vi "DiHuiTech Main.vi"(8 "error in (no error)":errorcluster caption="错误输入（无错误）", 10 "枚举":T3, 11 "Temperature&Humidity":T2) -> (0 "错误输出":errorcluster, 2 "value":T1, 3 "result":bool)   [LabVIEW 2017]
uses:
  DiHuiTech Operation.ctl
  DiHuiTech Param.ctl
  DiHuiTech Value.ctl
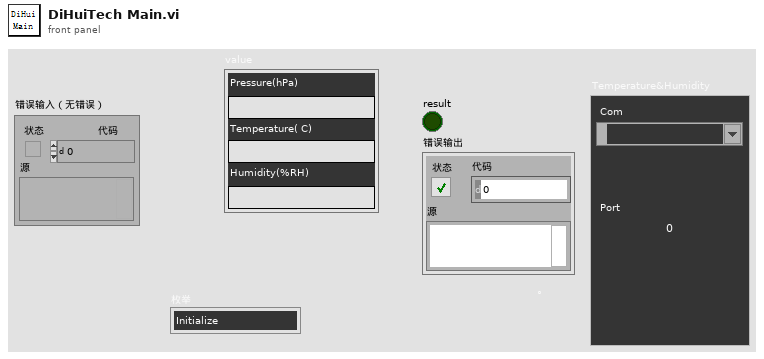
[diagram p1: front panel]
types:
  T1 = typedef "DiHuiTech Value.ctl" = cluster{"Pressure(hPa)":string, "Temperature( C)":string, "Humidity(%RH)":string}
  T2 = typedef "DiHuiTech Param.ctl" = cluster{"Com":refnum<visa-resource-name>, "Port":u32}
  T3 = typedef "DiHuiTech Operation.ctl" = enum16{"Initialize", "Read", "Exit"}
  T4 = cluster{"Pressure":dbl, "Temperature":dbl, "Humidity":dbl}
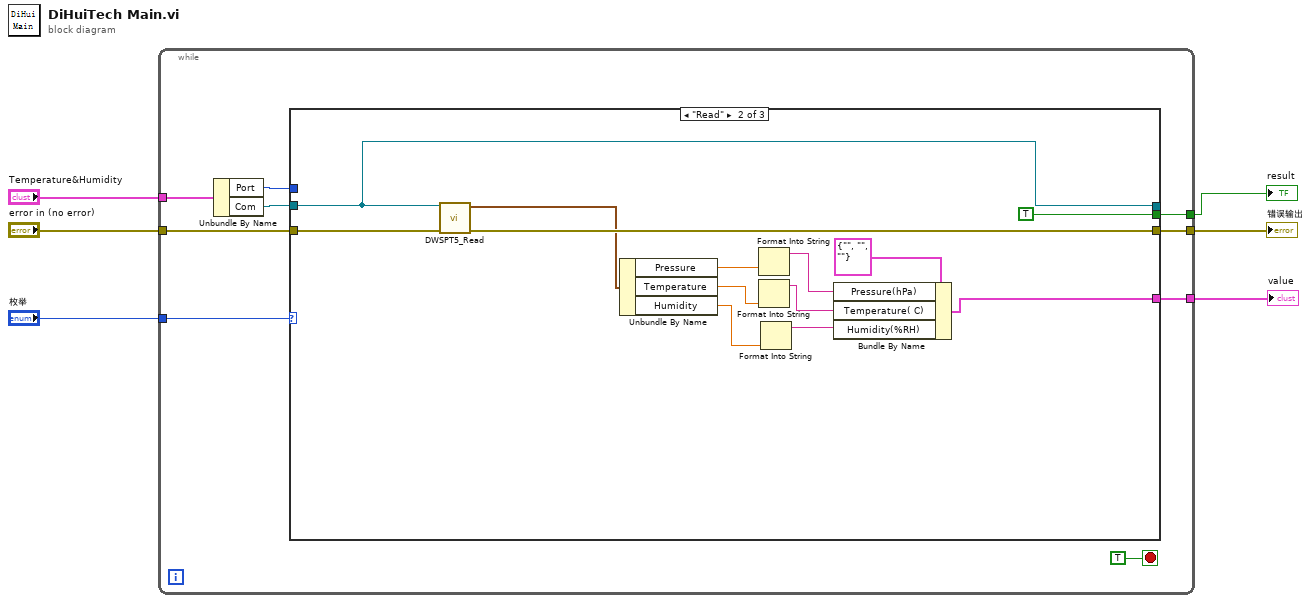
[diagram p0: block diagram]
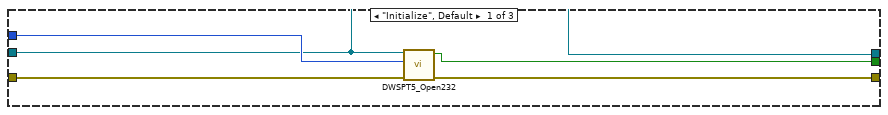
[diagram p2: hidden frame]
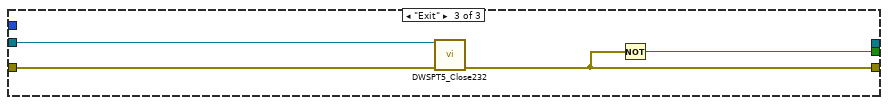
[diagram p3: hidden frame]
diagram:
  n1 = while {
    tunnel: "枚举" -> [w14]
    tunnel: [w13] -> w5
    tunnel: [w12] -> w4
    tunnel: "error in (no error)" -> [w11]
    tunnel: "Temperature&Humidity" -> [w7]
    tunnel: [w10] -> w1
    stop <- TRUE stop-if-true
    n2 = Unbundle By Name(w7) -> ("Port"=w8:u32, "Com"=w9:refnum<visa-resource-name>)
    n3 = case shown="\"Read\"" w14 {
      tunnel: [w17 w31 _] -> _
      tunnel: [w18 TRUE ("result") w37] -> w13
      tunnel: [w16 w30 w34] -> w12
      tunnel: w11 -> [w19 w32 w35]
      tunnel: w9 -> [w17 w31 w36]
      tunnel: [_ w28 _] -> w10
      tunnel: w8 -> [w20 _ _]
      frame "Initialize", Default {
        n4 = call "DWSPT5_Open232.vi"("error in (no error)"=w19, "baud rate (9600)"=w20, "VISA resource name"=w17) -> ("error out"=w16:errorcluster, "status"=w18:bool)  [unwired: 7 in]
      }
      frame "Read" {
        n5 = call "DWSPT5_Read.vi"("错误输入（无错误）"=w32, "VISA resource name"=w31) -> ("error out"=w30:errorcluster, "Data"=w27:T4)  [unwired: 8 in]
        n6 = Unbundle By Name(w27) -> ("Pressure"=w26:dbl, "Temperature"=w24:dbl, "Humidity"=w22:dbl)
        n7 = Format Into String(w26) -> (resulting string=w25:string)  [unwired: 3 in, 1 out]
        n8 = Format Into String(w24) -> (resulting string=w23:string)  [unwired: 3 in, 1 out]
        n9 = Format Into String(w22) -> (resulting string=w21:string)  [unwired: 3 in, 1 out]
        n10 = Bundle By Name(cluster=T1 {"Pressure(hPa)"="", "Temperature( C)"="", "Humidity(%RH)"=""} ("value"), "Pressure(hPa)"=w25, "Temperature( C)"=w23, "Humidity(%RH)"=w21) -> (w28:T1)
      }
      frame "Exit" {
        n11 = call "DWSPT5_Close232.vi"("error in (no error)"=w35, "VISA resource name"=w36) -> ("error out"=w34:errorcluster)  [unwired: 9 in]
        n12 = Not(x=w34) -> (.not. x?=w37:bool)
      }
    }
  }
  "result" <- w5
  "错误输出" <- w4
  "value" <- w1
